vi "CleanClose.vi"(8 "error in (no error)":errorcluster, 11 "Channel Manager in":refnum<class "Channel Manager.lvclass">) -> (0 "error out":errorcluster, 3 "Channel Manager out":refnum<class "Channel Manager.lvclass">)   [LabVIEW 2024, in "Embedded TDMS Logger Engine.lvlib" / "Channel Manager.lvclass"]
doc: "Cleanly closes the TDMS file currently in use and defragments it to reduce file sizes."
uses:
  Channel Manager.lvclass
  Channel Manager.lvclass/Channel Manager.ctl
  Shared/File Classes/File/File.lvclass
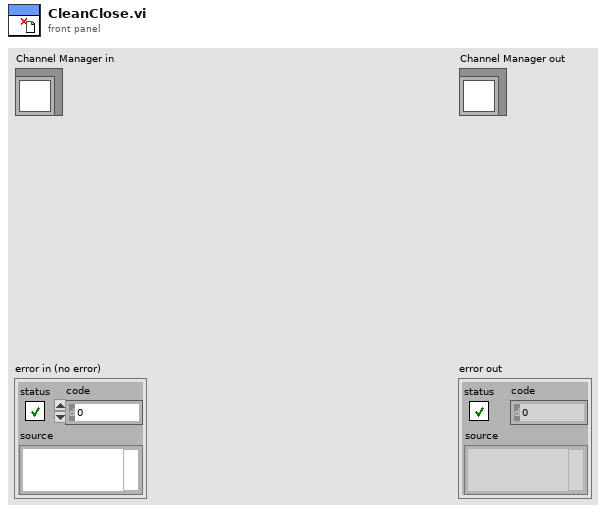
[diagram p1: front panel]
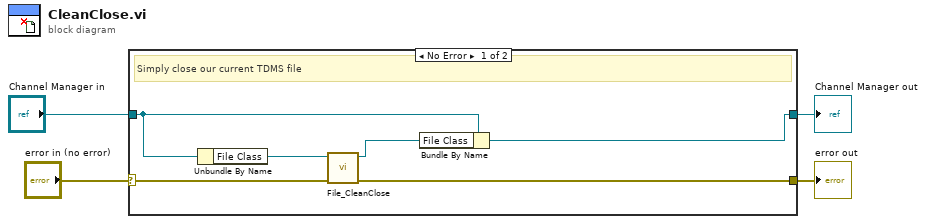
[diagram p0: block diagram]
diagram:
  n1 = case shown="No Error" "error in (no error)" {
    selector: "error in (no error)" -> [w5 w12]
    tunnel: [w6 w12] -> w3
    tunnel: [w8 w11] -> w1
    tunnel: "Channel Manager in" -> [w10 w11]
    frame No Error {
      # "Simply close our current TDMS file"
      n2 = Unbundle By Name(w10) -> ("File Class"=w9:refnum<class "File.lvclass">)
      n3 = call-dynamic "File_CleanClose.vi"("error in (no error)"=w5, "File in"=w9) -> ("error out"=w6:errorcluster, "File out"=w7:refnum<class "File.lvclass">)  [unwired: 8 in]
      n4 = Bundle By Name(cluster=w10, "File Class"=w7) -> (w8:refnum<class "Channel Manager.lvclass">)
    }
    frame Error {
    }
  }
  "error out" <- w3
  "Channel Manager out" <- w1
